vi "Integral Power BAP5.vi"(8 "Control Parameters":T1 {"Settle time" format="%.2f"; "Derivative time" format="%.2f"; "Integral time" format="%.2f"; "Settle bandwidth" format="%.2f"; "Control bandwidth" format="%.2f"; "Setpoint" format="%.2f"}, 9 "RESET":bool, 10 "elapsed time":dbl, 11 "Temp in (deg C)":dbl format="%#_13g") -> (3 "Integral Power":dbl)   [LabVIEW 2014]
doc: "Integral Power BAP5\n\nCalculates the Integral Power based off of Current Temperature (°C), Control Bandwidth (°C), Setpoint (°C), Integral Time (s), Elapsed Time (s), Counter, Integral On, and RESET. RESET initializes the Integral Power and Counter to 0.\n\nIntegral Power = Previous Integral Power - ((Current Temperature - Setpoint) * Elapsed Time) / (Control Bandwidth* Integral Time), if Integral On = True, and is within the control band.\n = 0, if Integral On = False, or Counter is greater than 1.\n\nBeverly Abadines \nPHY 350"
uses:
  typedefs/control parameters.ctl
panel:
  in  "Counter (k)":dbl format="%#_13g"
  # "Integral Power"
  # "Beverly Abadines\nPhys 350\nP5"
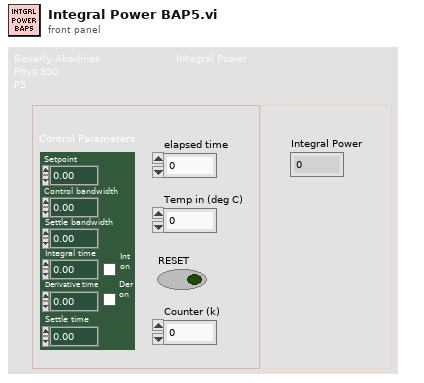
[diagram p1: front panel]
types:
  T1 = typedef "control parameters.ctl" = cluster{"Setpoint":dbl, "Control bandwidth":dbl, "Settle bandwidth":dbl, "Integral time":dbl, "Int\non":bool, "Derivative time":dbl, "Der\non":bool, "Settle time":dbl}
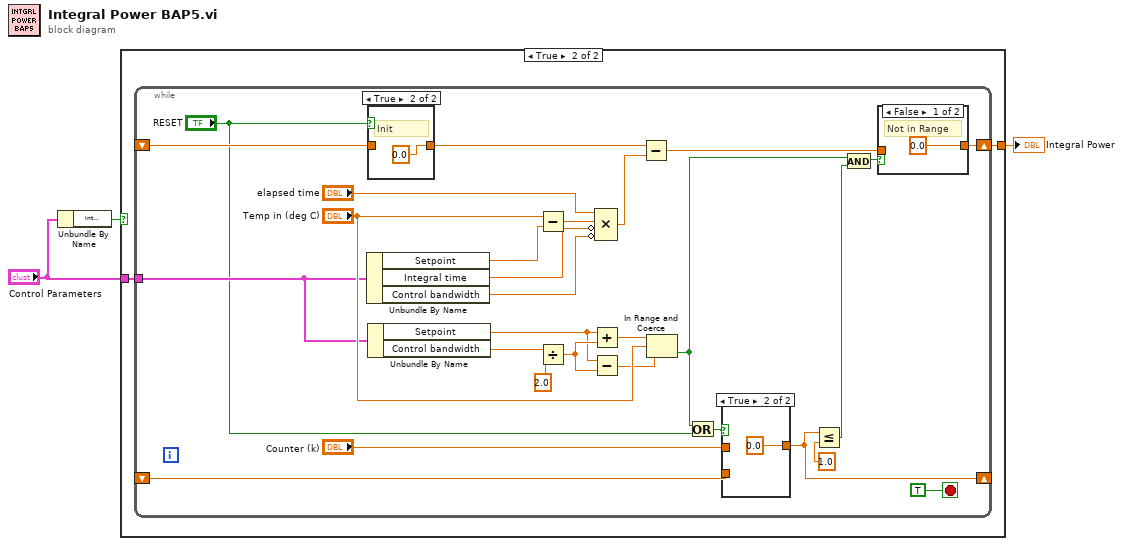
[diagram p0: block diagram]
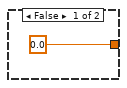
[diagram p2: hidden frame]
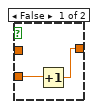
[diagram p3: hidden frame]
diagram:
  n1 = Unbundle By Name("Control Parameters") -> ("Int\non"=w2:bool)
  n2 = case shown="True" w2 {
    tunnel: [0.0 w6] -> w3
    tunnel: "Control Parameters" -> [_ w5]
    frame False {
    }
    frame True {
      n3 = while {
        shift-right: [w19] -> w6
        shift-left: _ -> [w28]
        tunnel: w5 -> [w18]
        shift-right: [w13] -> _
        shift-left: _ -> [w14]
        stop <- TRUE stop-if-true
        n4 = Unbundle By Name(w18) -> ("Setpoint"=w27:dbl, "Integral time"=w32:dbl, "Control bandwidth"=w26:dbl)
        n5 = case shown="True" "RESET" {
          tunnel: [w40 0.0] -> w31
          tunnel: w28 -> [w40 _]
          frame False {
          }
          frame True {
            # "Init"
          }
        }
        n6 = Unbundle By Name(w18) -> ("Setpoint"=w16:dbl, "Control bandwidth"=w17:dbl)
        n7 = Subtract(x="Temp in (deg C)", y=w27) -> (x-y=w34:dbl)
        n8 = Divide(x=w17, y=2.0) -> (x/y=w24:dbl)
        n9 = Add(x=w16, y=w24) -> (x+y=w22:dbl)
        n10 = Subtract(x=w16, y=w24) -> (x-y=w21:dbl)
        n11 = Compound Arithmetic op=MULTIPLY("elapsed time", w34, invert w32, invert w26) -> (w30:dbl)
        n12 = Subtract(x=w31, y=w30) -> (x-y=w20:dbl)
        n13 = In Range and Coerce(upper limit=w22, x="Temp in (deg C)", lower limit=w21) -> (In Range?=w8:bool)  [unwired: 1 out]
        n14 = Or(x=w8, y="RESET") -> (x .or. y?=w9:bool)
        n15 = case shown="True" w9 {
          tunnel: "Counter (k)" -> [_ _]
          tunnel: [w35 0.0] -> w13
          tunnel: w14 -> [w36 _]
          frame False {
            n16 = Increment(x=w36) -> (x+1=w35:dbl)
          }
          frame True {
          }
        }
        n17 = Less Or Equal?(x=w13, y=1.0) -> (x <= y?=w10:bool)
        n18 = And(x=w8, y=w10) -> (x .and. y?=w11:bool)
        n19 = case shown="False" w11 {
          tunnel: w20 -> [_ w39]
          tunnel: [0.0 w39] -> w19
          frame False {
            # "Not in Range"
          }
          frame True {
            # "W/in Range"
          }
        }
      }
    }
  }
  "Integral Power" <- w3
